vi "Change Endianness (U16).vi"(11 "number in":u16) -> (3 "byte-reversed number out":u16)   [LabVIEW 2016, in "GE 5565PIORC Old.lvclass"]
uses:
  GE 5565PIORC Old.lvclass
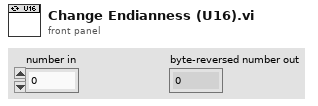
[diagram p1: front panel]
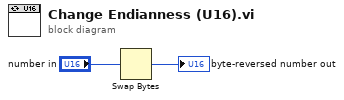
[diagram p0: block diagram]
diagram:
  n1 = Swap Bytes(anything="number in") -> (byte swapped=→"byte-reversed number out":u16)
